vi "CoboltLaser_AutostartStateSet.vi"(0 "ComPort":refnum<visa-resource-name>, 1 "AutostartEnable":bool=TRUE, 3 "CheckResponse":bool=TRUE, 7 "error in (no error)":errorcluster) -> (20 "ComPortOut":refnum<visa-resource-name>, 27 "error out":errorcluster)   [LabVIEW 2012, in "Cobolt.lvclass"]
doc: "Use this template to build a VI to use as a subVI."
uses:
  Template/Cobolt.lvclass
panel:
  out "ResponseOK":bool
  out "Response":string
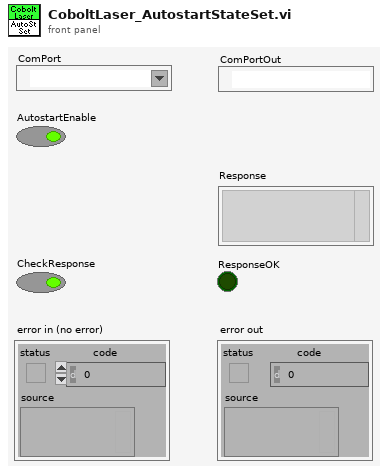
[diagram p1: front panel]
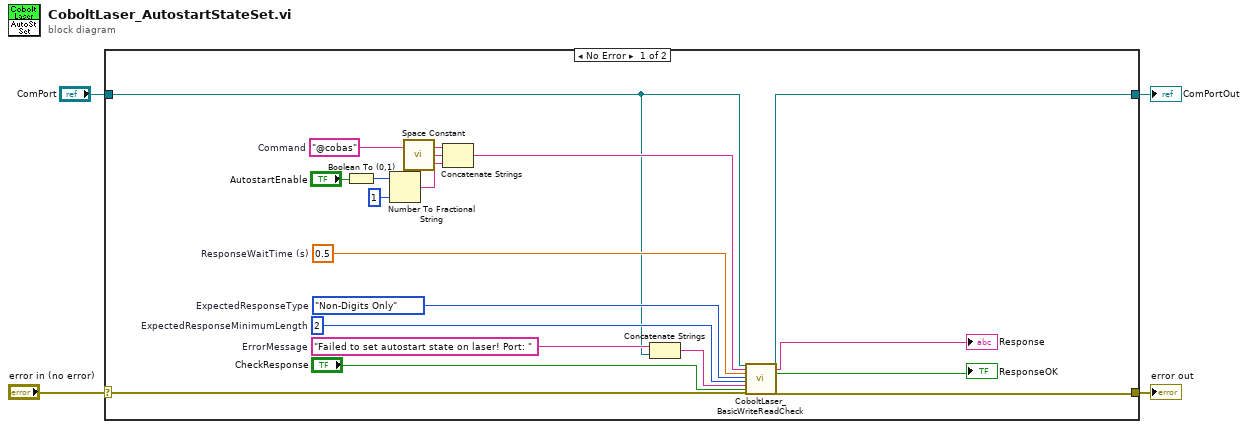
[diagram p0: block diagram]
diagram:
  n1 = case shown="No Error" "error in (no error)" {
    selector: "error in (no error)" -> [w23 w25]
    tunnel: [w22 w25] -> w3
    tunnel: "ComPort" -> [w6 w24]
    tunnel: [w5 w24] -> w1
    frame No Error {
      w19 = 2  # ExpectedResponseMinimumLength
      w20 = enum16{"Any", "Digits Only", "Non-Digits Only"}."Non-Digits Only"  # ExpectedResponseType
      w21 = 0.5  # ResponseWaitTime (s)
      w16 = "Failed to set autostart state on laser! Port: "  # ErrorMessage
      w10 = "@cobas"  # Command
      n2 = Boolean To (0,1)(Boolean="AutostartEnable") -> (0, 1=w7:i16)
      n3 = Number To Fractional String(number=w7, precision (6)=i16 1) -> (F-format string=w12:string)  [unwired: 2 in]
      n4 = call <vilib>:"Space Constant.vi"() -> ("String"=w13:string)
      n5 = Concatenate Strings(w10, w13, w12) -> (w9:string)
      n6 = Concatenate Strings(w16, w6) -> (w15:string)
      n7 = call "CoboltLaser_BasicWriteReadCheck.vi"("ComPort"=w6, "Command"=w9, "ResponseWaitTime (s)"=w21, "ExpectedResponseType"=w20, "ExpectedResponseMinimumLength"=w19, "ErrorMessage"=w15, "CheckResponse"="CheckResponse", "error in (no error)"=w23) -> ("ComPortOut"=w5:refnum<visa-resource-name>, "Response"=→"Response":string, "ResponseOK"=→"ResponseOK":bool, "error out"=w22:errorcluster)  [unwired: 16 in]
    }
    frame Error {
    }
  }
  "error out" <- w3
  "ComPortOut" <- w1
